vi "Changes Constant Types.vi"(5 "Requested Data Type":T1, 6 "Assert VI Path":path, 7 "String Control Name":string, 8 "error in (no error)":errorcluster) -> (0 "error out":errorcluster)   [LabVIEW 2016]
doc: "Updates the data types of required constants from the template block diagram in order to match the required assert functionality"
uses:
  <vilib>/Utility/Data Type/Type Definitions/Data Type.ctl
  <vilib>/Utility/Data Type/NI_Data Type.lvlib
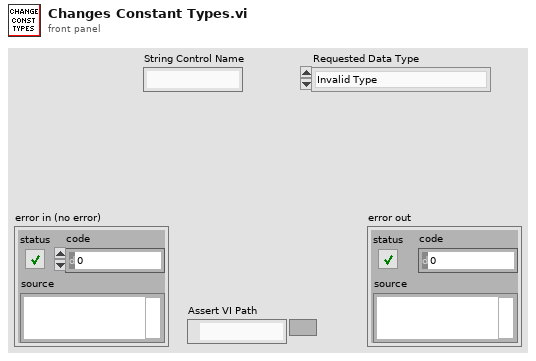
[diagram p1: front panel]
types:
  T1 = typedef "NI_Data Type.lvlib/Data Type.ctl" = enum8{"Invalid Type", "Void", "I8", "I16", "I32", "I64", "U8", "U16", "U32", "U64", "Single Float", "Double Float", "Extended Float", "Single Complex", "Double Complex", "Extended Complex", "Enum U8", "Enum U16", "Enum U32", "Enum U64", "Single Float With Unit", "Double Float With Unit", "Extended Float With Unit", "Single Complex with Unit", "Double Complex with Unit", "Extended Complex with Unit", "Boolean", "String", "Path", "Picture", "Tag", "Array", "Cluster", "Variant", "LV Variant", "Waveform", "Timestamp", "Digital Waveform", "Digital Data", "ExpressData", "Refnum", "External Data", "VI", "Poly VI", "LabVIEW Class Instance", "Fixed Point"}
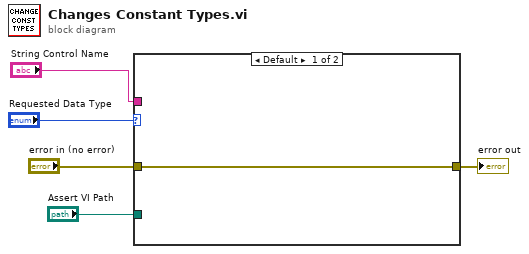
[diagram p0: block diagram]
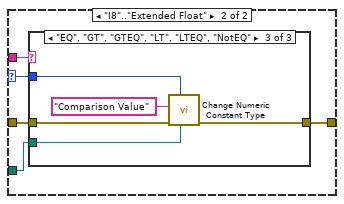
[diagram p2: hidden frame]
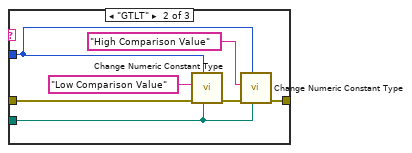
[diagram p4: hidden frame]
diagram:
  n1 = case shown="Default" "Requested Data Type" {
    selector: "Requested Data Type" -> [_ w10]
    tunnel: "error in (no error)" -> [w6 w11]
    tunnel: "String Control Name" -> [_ w9]
    tunnel: "Assert VI Path" -> [_ w8]
    tunnel: [w6 w7] -> w1
    frame Default {
    }
    frame "I8".."Extended Float" {
      n2 = case shown="\"EQ\", \"GT\", \"GTEQ\", \"LT\", \"LTEQ\", \"NotEQ\"" w9 {
        tunnel: w10 -> [_ w17 w23]
        tunnel: w8 -> [_ w16 w22]
        tunnel: w11 -> [w12 w15 w21]
        tunnel: [w12 w13 w20] -> w7
        frame Default {
        }
        frame "GTLT" {
          n3 = call "Change Numeric Constant Type.vi"("VI Path"=w16, "Data Type"=w17, "error in (no error)"=w15, "Control Name"="Low Comparison Value" ("Constant Name")) -> ("error out"=w14:errorcluster)  [unwired: 7 in]
          n4 = call "Change Numeric Constant Type.vi"("VI Path"=w16, "Data Type"=w17, "error in (no error)"=w14, "Control Name"="High Comparison Value" ("Constant Name")) -> ("error out"=w13:errorcluster)  [unwired: 7 in]
        }
        frame "EQ", "GT", "GTEQ", "LT", "LTEQ", "NotEQ" {
          n5 = call "Change Numeric Constant Type.vi"("VI Path"=w22, "Data Type"=w23, "error in (no error)"=w21, "Control Name"="Comparison Value" ("Constant Name")) -> ("error out"=w20:errorcluster)  [unwired: 7 in]
        }
      }
    }
  }
  "error out" <- w1
